vi "pr1c1.vi"() -> ()   [LabVIEW 2013]
uses:
  <vilib>/DAQmx/write.llb/DAQmx Write (Counter Frequency 1Chan 1Samp).vi
  <vilib>/platform/TimedLoop/XDataNode/XDataNode.xnode
  <vilib>/Platform/TimedLoop/XDataNode/timing_clust.ctl
  <vilib>/Platform/TimedLoop/XDataNode/XDNodeRunTimeDep.lvlib
  <vilib>/Platform/TimedLoop/XDataNode/wakeup.ctl
  <vilib>/Platform/TimedLoop/XDataNode/nitl_modes.ctl
  <vilib>/DAQmx/configure/timing.llb/DAQmx Timing (Implicit).vi
  <vilib>/DAQmx/create/channels.llb/DAQmx Create Channel (CO-Pulse Generation-Frequency).vi
panel:
  in  "x 2":dbl
  out "duty cicle ajustado":dbl
  in  "x":dbl
  in  "idle state":i32(ring)=10214 items=["High"=10192, "Low"=10214]
  in  "initial delay":dbl format="%.6f"
  in  "counter":tag
  in  "frequency":dbl=1.0 format="%.6f"
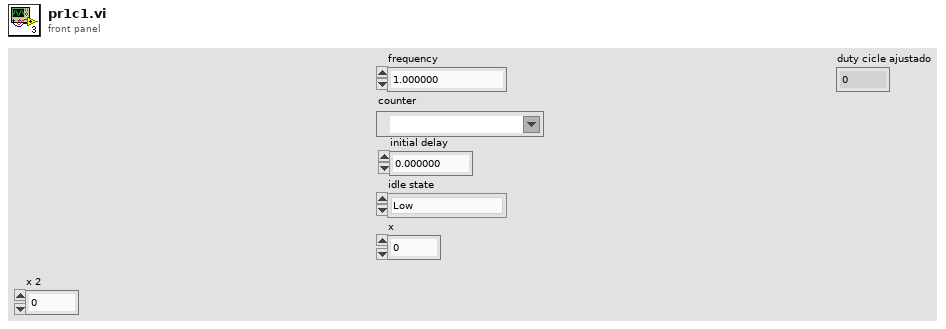
[diagram p1: front panel]
types:
  T1 = typedef "XDNodeRunTimeDep.lvlib/timing_clust.ctl" = cluster{"Expected End [f-1]":u64, "Actual End [f-1]":u64, "Finished Late? [f-1]":bool, "Expected End [i-1]":u64, "Actual End [i-1]":u64, "Finished Late? [i-1]":bool, "Expected Start [i]":u64, "Actual Start [i]":u64, "Expected Start [f]":u64, "Actual Start [f]":u64, "Source Name":string, "Structure Name":string, "Period":i64, "Deadline":i64, "Offset":i64, "Start":i64, "Priority":i32, "Timeout":i32, "Mode":T2, "Wakeup Reason":T3, "Error":errorcluster, "Source Type":string, "Secondary Source Type":string, "Global End Time":u64, "Global Start Time":u64, "Frame Duration":u64, "Iteration Duration":u64, "Assigned CPU":i32, "I/O Scan Engine Mode":u32}
  T2 = typedef "XDNodeRunTimeDep.lvlib/nitl_modes.ctl" = enum32{"No Change", "Process missed periods, maintain original phase", "Discard missed periods, maintain original phase", "Process missed periods, ignore original phase", "Discard missed periods, ignore original phase"}
  T3 = typedef "XDNodeRunTimeDep.lvlib/wakeup.ctl" = enum32{"Normal", "Aborted", "Asynchronous wakeup", "Timing source error", "Timed loop error", "Timeout"}
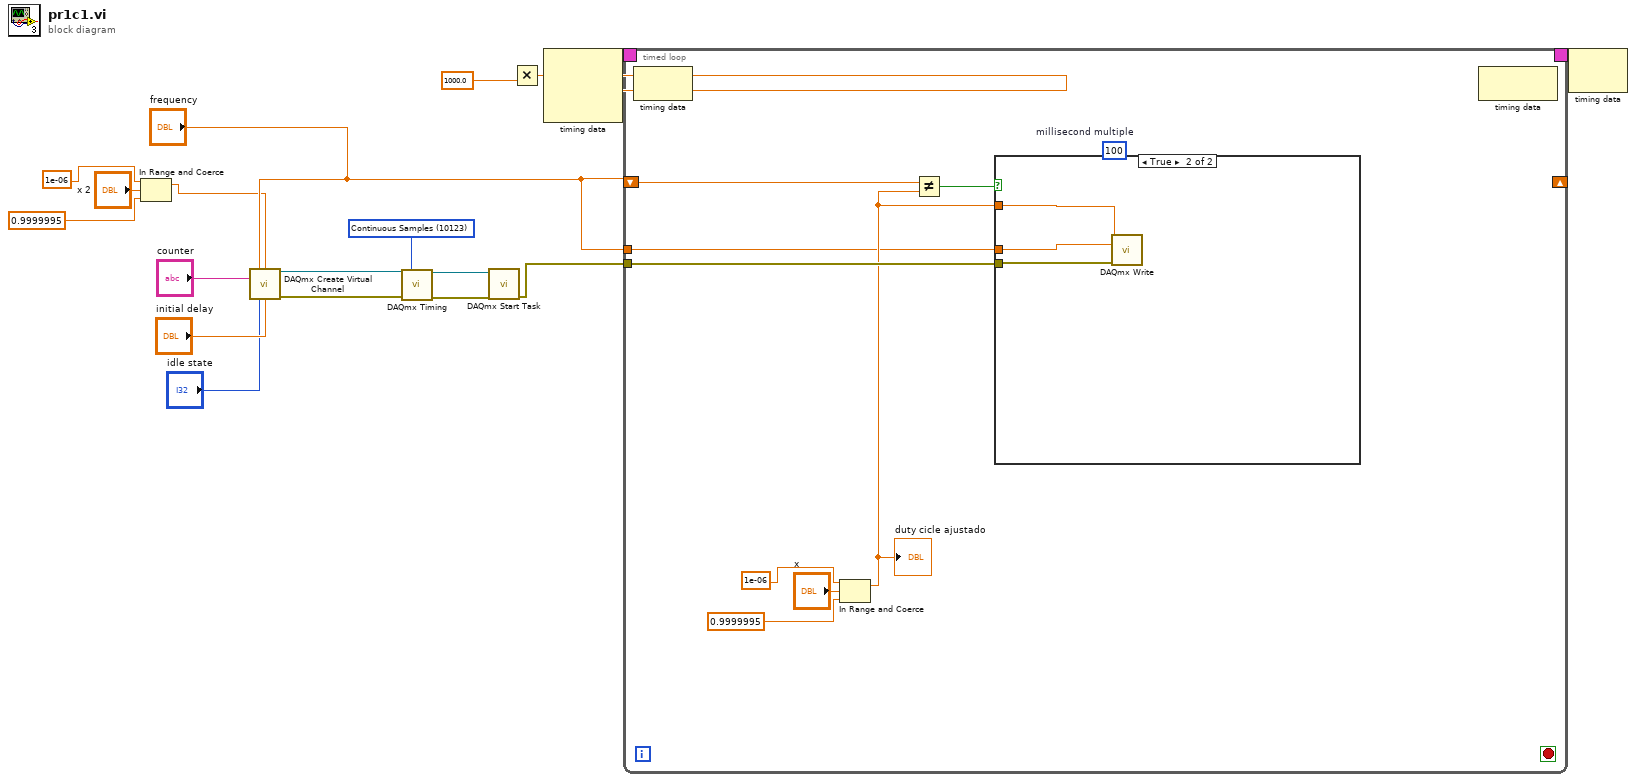
[diagram p0: block diagram]
diagram:
  w16 = 10123 items=["Finite Samples"=10178, "Continuous Samples"=10123, "Hardware Timed Single Point"=12522] ("sample mode")
  (unwired) u32 100  # millisecond multiple
  n1 = In Range and Coerce(upper limit=1e-06, x="x 2", lower limit=0.9999995 ("x")) -> (coerced(x)=w1:dbl)  [unwired: 1 out]
  n2 = call-poly <vilib>:"DAQmx Create Virtual Channel.vi"("frequency"="frequency", "duty cycle"=w1, "counter"="counter", "idle state"="idle state", "initial delay"="initial delay") -> ("task out"=w18:refnum<k21>, "error out"=w17:errorcluster)  [unwired: 9 in]
  n3 = call-poly <vilib>:"DAQmx Timing.vi"("task/channels in"=w18, "sample mode"=w16, "error in"=w17) -> ("task out"=w15:refnum<k21>, "error out"=w14:errorcluster)  [unwired: 11 in]
  n4 = call <vilib>:"DAQmx Start Task.vi"("task/channels in"=w15, "error in"=w14) -> ("error out"=w6:errorcluster)  [unwired: 12 in, 1 out]
  n5 = Multiply(y=1000.0) -> (x*y=w11:dbl)  [unwired: 1 in]
  n6 = node-c288(w11) -> (w13:T1)  [unwired: 2 in]
  n7 = timed-loop {
    timing: w13 -> [_]
    timing-out: [_] -> w12
    tunnel: w6 -> [w22]
    shift-right: _ -> [_]
    shift-left: "frequency" -> [w20]
    tunnel: "frequency" -> [w19]
    stop <- _ stop-if-true
    n8 = node-c288() -> ()  [unwired: 1 in, 1 out]
    n9 = In Range and Coerce(upper limit=1e-06, x="x", lower limit=0.9999995 ("x")) -> (coerced(x)=w21:dbl)  [unwired: 1 out]
    "duty cicle ajustado" <- w21
    n10 = Not Equal?(x=w20, y=w21) -> (x != y?=w26:bool)
    n11 = case shown="True" w26 {
      tunnel: w22 -> [_ w29]
      tunnel: w21 -> [_ w28]
      tunnel: w19 -> [_ w27]
      frame False {
      }
      frame True {
        n12 = call-poly <vilib>:"DAQmx Write.vi"("frequency"=w27, "duty cycle"=w28, "error in"=w29) -> ()  [unwired: 10 in, 3 out]
      }
    }
    n13 = node-c288() -> ()  [unwired: 1 in, 1 out]
  }
  n14 = node-c288(w12) -> ()  [unwired: 1 out]
